vi "Switch Configuration - Initialize ListBoxes.vi"(8 "error in (no error)":errorcluster, 9 "Channels ListBox Items":string[](array[string]), 10 "Selectable Channels ListBox Items":string[](array[string]), 11 "Switch Config UI Data In":T1 {"Switch Config Page Item Ref" format="%.0x"}) -> (0 "error out":errorcluster, 3 "Switch Config UI Data Out":T1 {"Switch Config Page Item Ref" format="%.0x"})   [LabVIEW 2015, in "DMM-SWITCH-ScanList System Explorer.lvlib"]
doc: "Copies current Channel Array from Origin ListBox to Destiny ListBox and deletes Channel Array from Origin ListBox afterwards."
uses:
  DMM-SWITCH-ScanList System Explorer.lvlib
  Configuration Controls/Switch Config VI UI Data.ctl
  Configuration Controls/Switch Config VI UI Ctrl Values.ctl
  Configuration Controls/Switch Config VI UI Ctrl References.ctl
  <instrlib>/niSwitch/niSwitch.LLB/niSwitch Topologies.ctl
  <vilib>/NI Veristand/Custom Device API/Custom Device Item Ref.ctl
  <vilib>/NI Veristand/Custom Device API/Custom Device API.lvlib
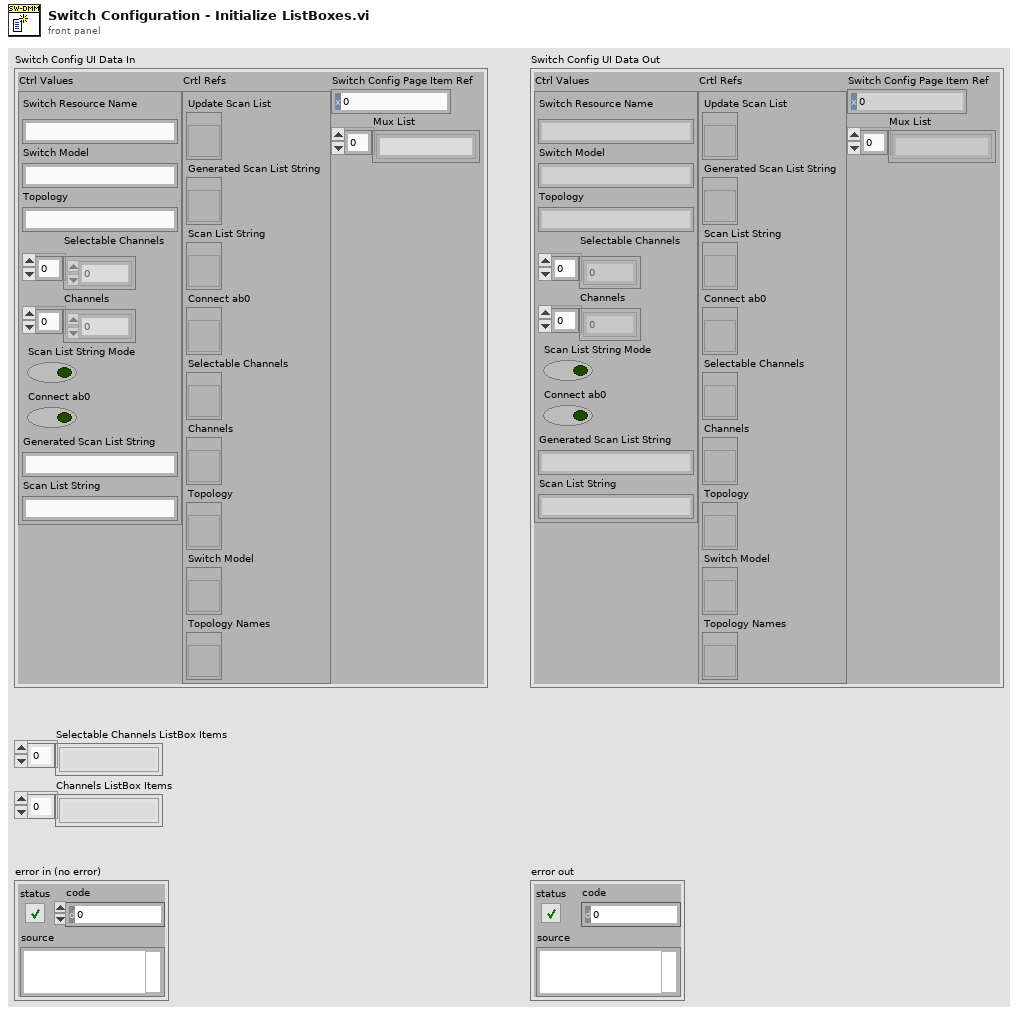
[diagram p1: front panel]
types:
  T1 = typedef "DMM-SWITCH-ScanList System Explorer.lvlib/Switch Config VI UI Data.ctl" = cluster{"Ctrl Values":T2, "Crtl Refs":T3, "Switch Config Page Item Ref":T4, "Mux List":string[]}
  T2 = typedef "DMM-SWITCH-ScanList System Explorer.lvlib/Switch Config VI UI Ctrl Values.ctl" = cluster{"Switch Resource Name":string, "Switch Model":string, "Topology":string, "Selectable Channels":i32[], "Channels":i32[], "Scan List String Mode":bool, "Connect ab0":bool, "Generated Scan List String":string, "Scan List String":string}
  T3 = typedef "DMM-SWITCH-ScanList System Explorer.lvlib/Switch Config VI UI Ctrl References.ctl" = cluster{"Update Scan List":refnum<vi>, "Generated Scan List String":refnum<vi>, "Scan List String":refnum<vi>, "Connect ab0":refnum<vi>, "Selectable Channels":refnum<vi>, "Channels":refnum<vi>, "Topology":refnum<vi>, "Switch Model":refnum<vi>, "Topology Names":refnum<vi>}
  T4 = typedef "Custom Device API.lvlib/Custom Device Item Ref.ctl" = u64
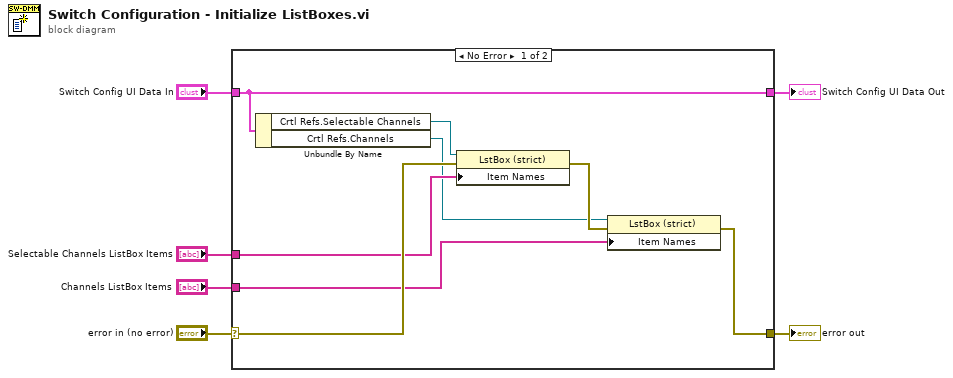
[diagram p0: block diagram]
diagram:
  n1 = case shown="No Error" "error in (no error)" {
    selector: "error in (no error)" -> [w12 w16]
    tunnel: [w14 w16] -> w6
    tunnel: "Selectable Channels ListBox Items" -> [w11 _]
    tunnel: "Channels ListBox Items" -> [w10 _]
    tunnel: "Switch Config UI Data In" -> [w7 w15]
    tunnel: [w7 w15] -> w1
    frame No Error {
      n2 = Unbundle By Name(w7) -> ("Crtl Refs.Selectable Channels"=w8:refnum<vi>, "Crtl Refs.Channels"=w9:refnum<vi>)
      n3 = property class="LstBox (strict)"(reference=w8, error in=w12, "Item Names"=w11) -> (error out=w13:errorcluster)  [unwired: 1 out]
      n4 = property class="LstBox (strict)"(reference=w9, error in=w13, "Item Names"=w10) -> (error out=w14:errorcluster)  [unwired: 1 out]
    }
    frame Error {
    }
  }
  "error out" <- w6
  "Switch Config UI Data Out" <- w1
